vi "Register API.vi"(8 "error in (no error)":errorcluster, 10 "API":refnum<class "API.lvclass">, 11 "VolatusCore in":refnum<class "VolatusCoreTask.lvclass">) -> (0 "error out":errorcluster, 3 "VolatusCore out":refnum<class "VolatusCoreTask.lvclass">)   [LabVIEW 2020, in "Volatus.lvlib" / "VolatusCoreTask.lvclass"]
uses:
  VolatusCoreTask.lvclass
  API/API.lvclass
  VolatusCoreTask.lvclass/VolatusCoreTask.ctl
  <vilib>/Utility/miscctls.llb/LVMapReplaceAction.ctl
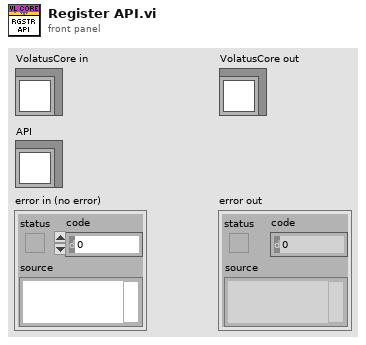
[diagram p1: front panel]
types:
  T1 = typedef "LVMapReplaceAction.ctl" = enum32{"Modify Entry only if found", "Add or Modify Entry", "Delete Entry"}
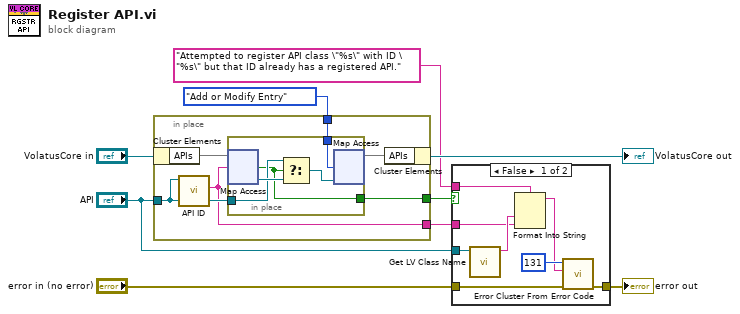
[diagram p0: block diagram]
diagram:
  n1 = in-place {
    in-place-border: "API" -> [w14]
    in-place-border: LVMapReplaceAction."Add or Modify Entry" ("action") -> [w13]
    in-place-border: [w11] -> w7
    in-place-border: [w10] -> w6
    n2 = in-place-cluster #1("VolatusCore in") -> ("APIs"=w15:map{string, refnum<class "API.lvclass">})
    n3 = call-dynamic "API ID.vi"("API in"=w14) -> ("ID"=w10:string)  [unwired: 10 in]
    n4 = in-place {
      in-place-border: w14 -> [w19]
      in-place-border: w13 -> [w17]
      in-place-border: [w16] -> w11
      n5 = in-place-map #2(w15, w10) -> (w20:refnum<class "API.lvclass">, w16:bool)  [unwired: 1 in]
      n6 = Select(t=w19, s=w16, f=w20) -> (s? t:f=w18:refnum<class "API.lvclass">)
      n7 = in-place-map #2(w18, w17) -> (w12:map{string, refnum<class "API.lvclass">})  [unwired: 2 out]
    }
    n8 = in-place-cluster #1("APIs"=w12) -> (→"VolatusCore out":refnum<class "VolatusCoreTask.lvclass">)
  }
  n9 = case shown="False" w7 {
    tunnel: w6 -> [w25 _]
    tunnel: "API" -> [w28 _]
    tunnel: "Attempted to register API class \"%s\" with ID \"%s\" but that ID already has a registered API." -> [w27 _]
    tunnel: [w22 w29] -> w2
    tunnel: "error in (no error)" -> [w21 w29]
    frame False {
      n10 = call <vilib>:"Get LV Class Name.vi"("object"=w28) -> ("class name"=w26:string)  [unwired: 9 in, 1 out]
      n11 = Format Into String(format string=w27, w26, w25) -> (resulting string=w23:string)  [unwired: 2 in, 1 out]
      n12 = call <vilib>:"Error Cluster From Error Code.vi"("error in (no error)"=w21, "error message (\"\")"=w23, "error code (0)"=131) -> ("error out"=w22:errorcluster)  [unwired: 6 in]
    }
    frame True {
    }
  }
  "error out" <- w2
